vi "5-4_FanControlWithLongPushImmediateStop.vi"() -> ()   [LabVIEW 2014]
doc: "This example demonstrates how to read one channel of digital input from a LINX device.\n------------------------------------\nAuther: Koji Ohashi\nCopyright (c) 2020 Japan LabVIEW Users Group, Volunteer members.\nThis VI is released under the MIT License.\nhttp://opensource.org/licenses/mit-license.php\n------------------------------------"
uses:
  <vilib>/MakerHub/LINX/LMH-LINX.lvlib
  <vilib>/MakerHub/LINX/Public/Peripherals/Digital/Digital Read 1 Chan.vi
  <vilib>/MakerHub/LINX/Public/Utilities/Open Serial.vi
  <vilib>/MakerHub/LINX/Public/Peripherals/PWM/PWM Set Duty Cycle 1 Chan.vi
panel:
  out "Running":bool
  in  "Hardware Setting":cluster{"SW":u8, "Fan":u8}={"SW"=8, "Fan"=9}
  out "Count":i32
  out "DI Value":bool
  in  "Stop Button":bool
  in  "Serial Port":refnum<visa-resource-name>
  # "LINX Device Settings"
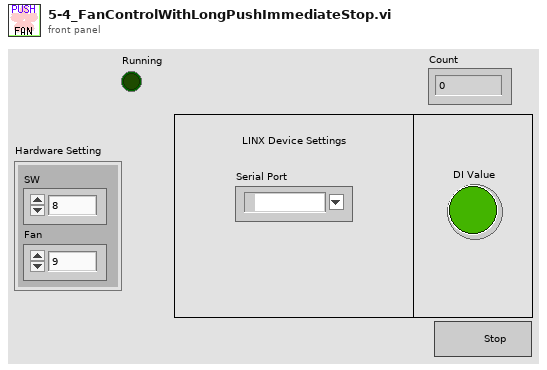
[diagram p1: front panel]
types:
  T1 = typedef "LMH-LINX.lvlib/LINX Ref.ctl" = cluster{"IO":T2, "Interface":T3, "LINX Device Config":T4}
  T2 = typedef "LMH-LINX.lvlib/Platform.ctl" = enum16{"Remote", "Local"}
  T3 = typedef "LMH-LINX.lvlib/Interface.ctl" = enum16{"Serial", "TCP"}
  T4 = typedef "LMH-LINX.lvlib/Device.lvlib/LINX Device Config.ctl" = cluster{"Interface":T3, "COM Port":refnum<visa-resource-name>, "TCP Configuration":T5, "Device Family":u8, "Device ID":u8, "Device Name":string, "TCP Ref":refnum<k5>, "Channels":T6}
  T5 = typedef "LMH-LINX.lvlib/Device.lvlib/TCP Config.ctl" = cluster{"IP Address":string, "Port":u16}
  T6 = typedef "LMH-LINX.lvlib/Channels.ctl" = cluster{"DI":u8[], "DO":u8[], "AI":u8[], "AO":u8[], "PWM":u8[], "QE":u8[], "UART":u8[], "I2C 2":u8[], "SPI":u8[], "CAN":u8[], "Servo":u8[], "AI Ref (V)":dbl, "AI Resolution (Bits)":u8, "AO Ref (V)":dbl, "AO Resolution (Bits)":u8}
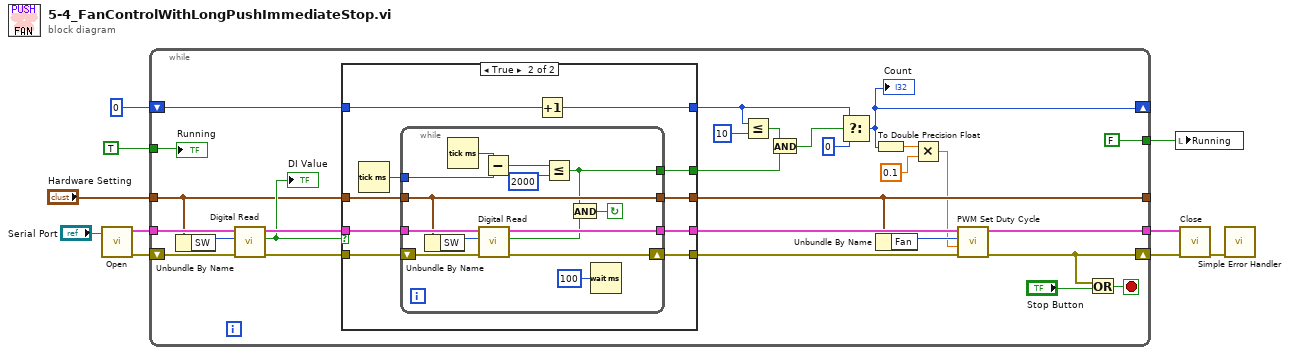
[diagram p0: block diagram]
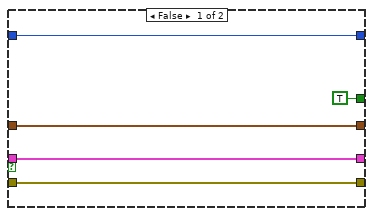
[diagram p2: hidden frame]
diagram:
  n1 = call-poly <vilib>:"Open.vi"("Serial Port"="Serial Port") -> ("Error Out"=w9:errorcluster, "LINX Resource"=w10:T1)  [unwired: 8 in, 1 out]
  n2 = while {
    tunnel: w10 -> [w36]
    tunnel: [w24] -> w8
    shift-right: [w26] -> w7
    shift-left: w9 -> [w35]
    tunnel: "Hardware Setting" -> [w23]
    shift-right: [w19] -> _
    shift-left: 0 -> [w30]
    tunnel: [w21] -> _
    tunnel: TRUE ("Running") -> [w12]
    tunnel: [FALSE ("Running")] -> w1
    stop <- w38 stop-if-true
    n3 = Unbundle By Name(w23) -> ("SW"=w22:u8)
    n4 = call-poly <vilib>:"Digital Read.vi"("Error In"=w35, "DI Channel"=w22, "LINX Resource"=w36) -> ("Error Out"=w31:errorcluster, "DI Value"=w28:bool, "LINX Resource"=w32:T1)  [unwired: 6 in]
    "DI Value" <- w28
    n5 = case shown="TRUE" w28 {
      tunnel: w32 -> [w41 w53]
      tunnel: w23 -> [w40 w52]
      tunnel: w31 -> [w43 w51]
      tunnel: [w43 w50] -> w27
      tunnel: w30 -> [w42 w47]
      tunnel: [w42 w49] -> w29
      tunnel: [w41 w48] -> w25
      tunnel: [w40 w46] -> w21
      tunnel: [TRUE w44] -> w15
      frame False {
      }
      frame True {
        n6 = Tick Count (ms)() -> (millisecond timer value=w45:u32)
        n7 = while {
          tunnel: w53 -> [w67]
          tunnel: w52 -> [w61]
          shift-right: [w65] -> w50
          shift-left: w51 -> [w66]
          tunnel: [w63] -> w48
          tunnel: [w61] -> w46
          tunnel: w45 -> [w59]
          tunnel: [w56] -> w44
          stop <- w54 continue-if-true
          n8 = Unbundle By Name(w61) -> ("SW"=w62:u8)
          n9 = Tick Count (ms)() -> (millisecond timer value=w60:u32)
          n10 = call-poly <vilib>:"Digital Read.vi"("Error In"=w66, "DI Channel"=w62, "LINX Resource"=w67) -> ("Error Out"=w65:errorcluster, "DI Value"=w55:bool, "LINX Resource"=w63:T1)  [unwired: 6 in]
          n11 = Subtract(x=w60, y=w59) -> (x-y=w58:u32)
          n12 = Less Or Equal?(x=w58, y=u32 2000) -> (x <= y?=w56:bool)
          n13 = And(x=w56, y=w55) -> (x .and. y?=w54:bool)
          n14 = Wait (ms)(milliseconds to wait=u32 100) -> ()  [unwired: 1 out]
        }
        n15 = Increment(x=w47) -> (x+1=w49:i32)
      }
    }
    n16 = Less Or Equal?(x=w29, y=10) -> (x <= y?=w14:bool)
    n17 = And(x=w14, y=w15) -> (x .and. y?=w13:bool)
    n18 = Select(t=w29, s=w13, f=0) -> (s? t:f=w19:i32)
    "Count" <- w19
    n19 = To Double Precision Float(number=w19) -> (double precision float=w17:dbl)
    n20 = Unbundle By Name(w21) -> ("Fan"=w20:u8)
    n21 = Multiply(x=w17, y=0.1) -> (x*y=w16:dbl)
    n22 = call-poly <vilib>:"PWM Set Duty Cycle.vi"("Error In"=w27, "Duty Cycle (0-1)"=w16, "PWM Channel"=w20, "LINX Resource"=w25) -> ("Error Out"=w26:errorcluster, "LINX Resource"=w24:T1)  [unwired: 6 in]
    n23 = Or(x=w26, y="Stop Button") -> (x .or. y?=w38:bool)
    "Running" <- w12
  }
  n24 = local write "Running"(w1) -> ()
  n25 = call <vilib>:"Close.vi"("Error In"=w7, "LINX Resource"=w8) -> ("Error Out"=w5:errorcluster)  [unwired: 9 in]
  n26 = call <vilib>:"Simple Error Handler.vi"("error in (no error)"=w5) -> ()  [unwired: 4 in, 5 out]
